vi "Read Data File.vi"() -> ()   [LabVIEW 2009]
panel:
  out "Signals":dynamicdata(graph)
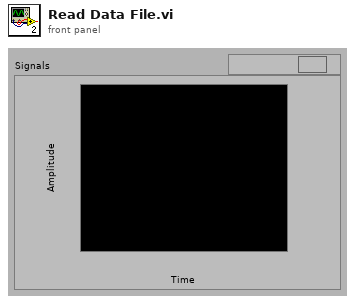
[diagram p1: front panel]
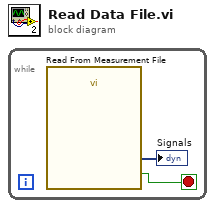
[diagram p0: block diagram]
diagram:
  n1 = while {
    stop <- w1 stop-if-true
    n2 = call "Read From Measurement File"() -> ("Signals"=→"Signals":dynamicdata, "EOF?"=w1:bool)  [unwired: 6 in, 4 out]
  }
